vi "process.vi"() -> ()   [LabVIEW 2019]
uses:
  drivers/evcxxx.lvlib
panel:
  out "Device":T1={"Name"="---", "Type"=enum."Standard", "Class"=0, "FW-Rev"=0.0, "HV max"=0.0, "Emis max"=0.0}
  out "Data Cluster #1":T2 {"Flux" format="%^#_6e"; "Fil" format="%.2f"; "Emis" format="%.1f"; "HV" format="%#.0f"}
  out "Data Cluster #2":T3 {"Aux" format="%.2f"; "Sample" format="%^#_6e"}
  out "Data Cluster #3":T4 {"Fil max" format="%.2f"; "Emis max" format="%.1f"}
  out "Data Cluster #4":T5={"TMR Start"="00:00:00", "TMR/CLK"="00:00:00", "Dep Start"=0.0, "Dep/Exp"=0.0} {"Dep/Exp" format="%^#_6e"; "Dep Start" format="%^#_6e"}
  out "Data Cluster #5":T6 {"Fil nom" format="%.2f"; "Emis nom" format="%.1f"}
  out "Data Cluster #6":cluster{"AU-SP":dbl, "FL-SP":dbl} {"FL-SP" format="%^#_6e"; "AU-SP" format="%.2f"}
  out "Data Cluster #7":T7
  out "Status":T8
  out "Shutter":T9
  in  "OK":bool
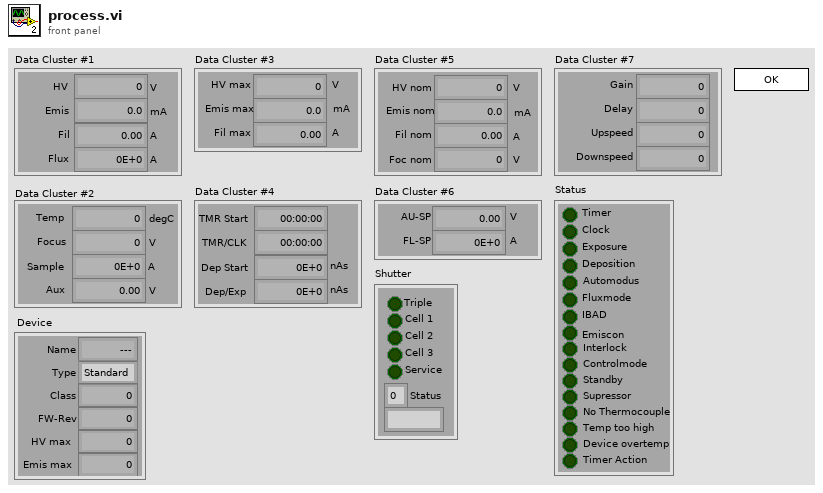
[diagram p1: front panel]
types:
  T1 = cluster{"Name":string, "Type":enum16{"Standard", "IBAD", "Supr"}, "Class":u16, "FW-Rev":dbl, "HV max":dbl, "Emis max":dbl}
  T2 = cluster{"HV":dbl, "Emis":dbl, "Fil":dbl, "Flux":dbl}
  T3 = cluster{"Temp":dbl, "Focus":dbl, "Sample":dbl, "Aux":dbl}
  T4 = cluster{"HV max":dbl, "Emis max":dbl, "Fil max":dbl}
  T5 = cluster{"TMR Start":string, "TMR/CLK":string, "Dep Start":dbl, "Dep/Exp":dbl}
  T6 = cluster{"HV nom":dbl, "Emis nom":dbl, "Fil nom":dbl, "Foc nom":dbl}
  T7 = cluster{"Gain":i32, "Delay":i32, "Upspeed":i32, "Downspeed":i32}
  T8 = cluster{"Timer":bool, "Clock":bool, "Exposure":bool, "Deposition":bool, "Automodus":bool, "Fluxmode":bool, "IBAD":bool, "Emiscon":bool, "Interlock":bool, "Controlmode":bool, "Standby":bool, "Supressor":bool, "No Thermocouple":bool, "Temp too high":bool, "Device overtemp":bool, "Timer Action":bool}
  T9 = cluster{"Triple":bool, "Cell 1":bool, "Cell 2":bool, "Cell 3":bool, "Service":bool, "iStatus":u8, "strStatus":string}
  T10 = enum32{"Invalid", "Standard", "Closed", "Hidden", "Minimized", "Maximized"}
  T11 = enum32{"invalid app kind", "Development System", "Run Time System", "Student Edition", "Embedded LabVIEW", "Evaluation", "Custom"}
  T12 = cluster{"Core":cluster{"Current VI Reference":refnum<vi>, "Close Panel on Exit?":bool}, "Your Boolean data":bool, "Your string data":string}
  T13 = cluster{"Current VI Reference":refnum<vi>, "Close Panel on Exit?":bool}
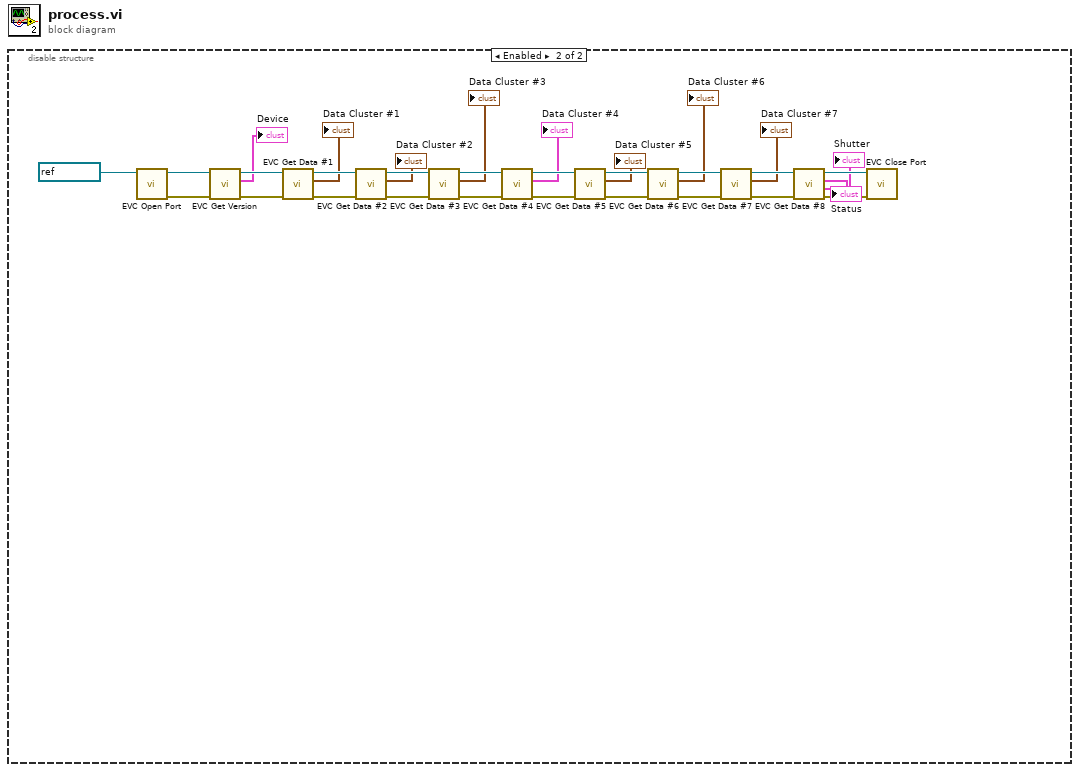
[diagram p0: block diagram]
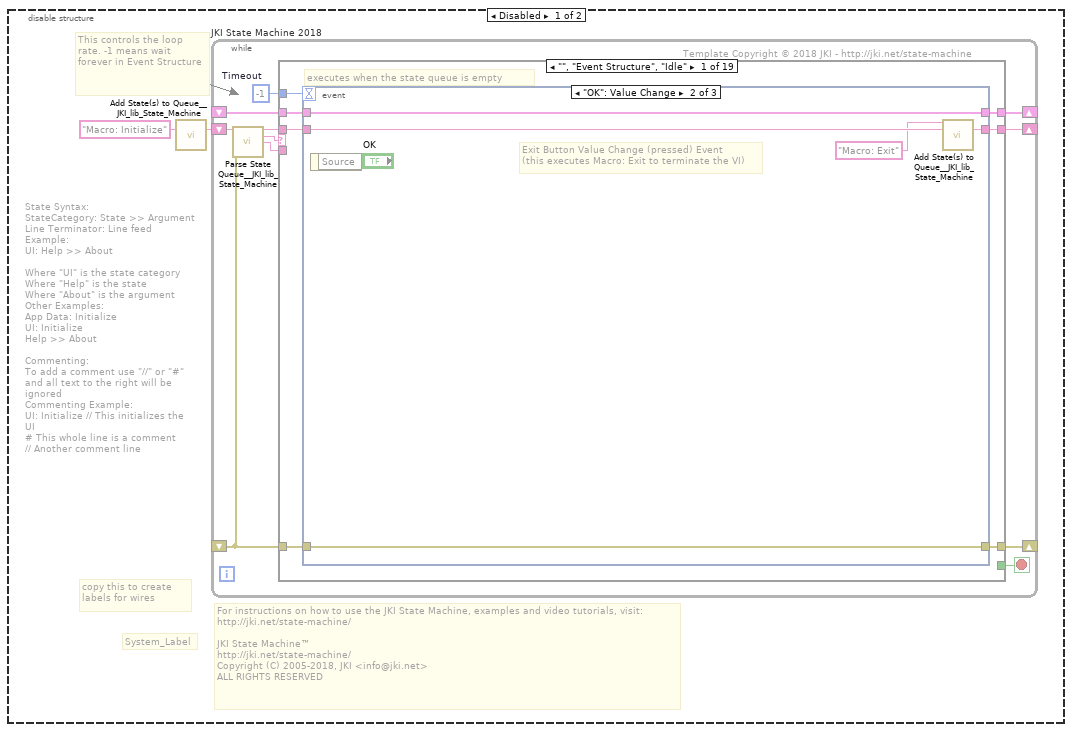
[diagram p2: hidden frame]
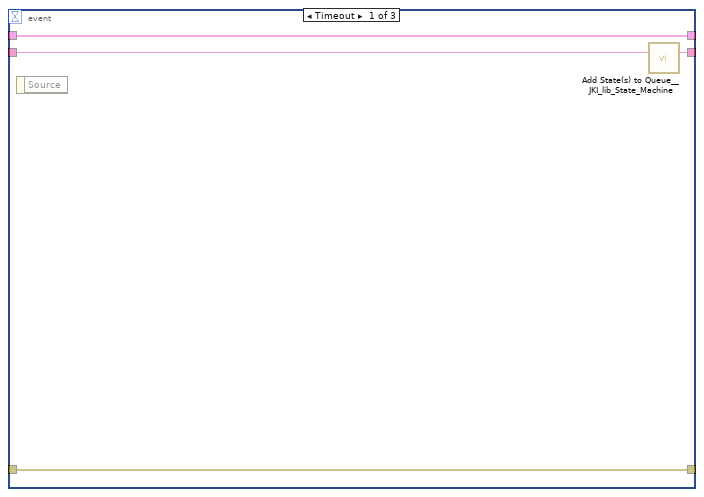
[diagram p3: hidden frame]
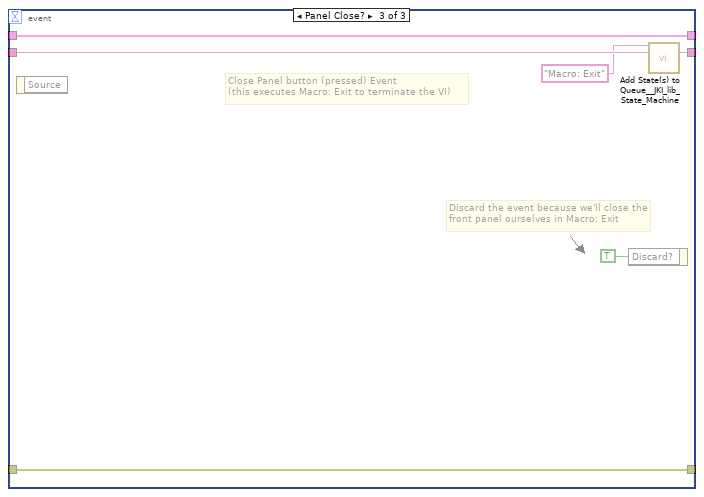
[diagram p4: hidden frame]
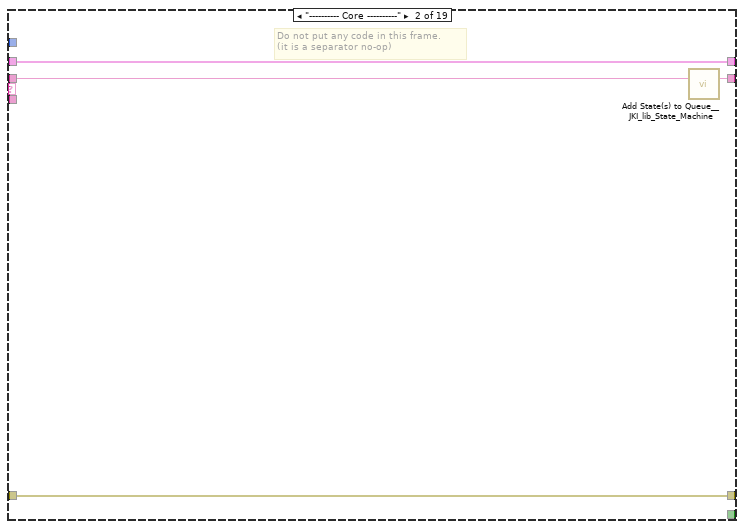
[diagram p5: hidden frame]
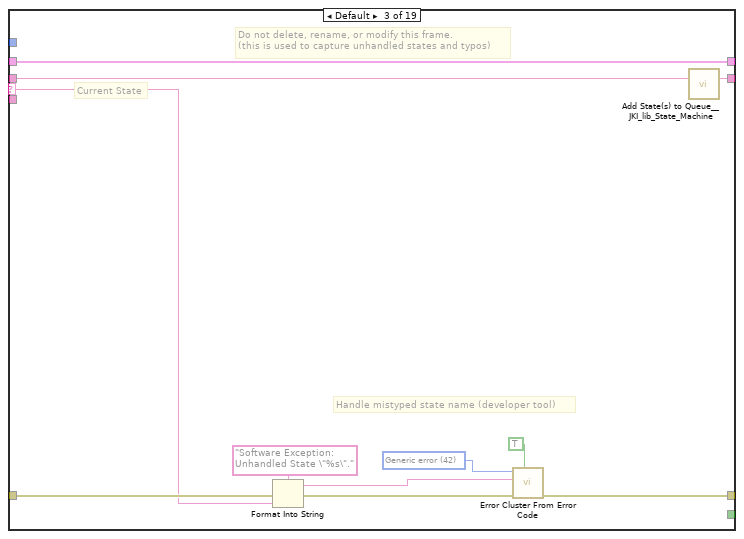
[diagram p6: hidden frame]
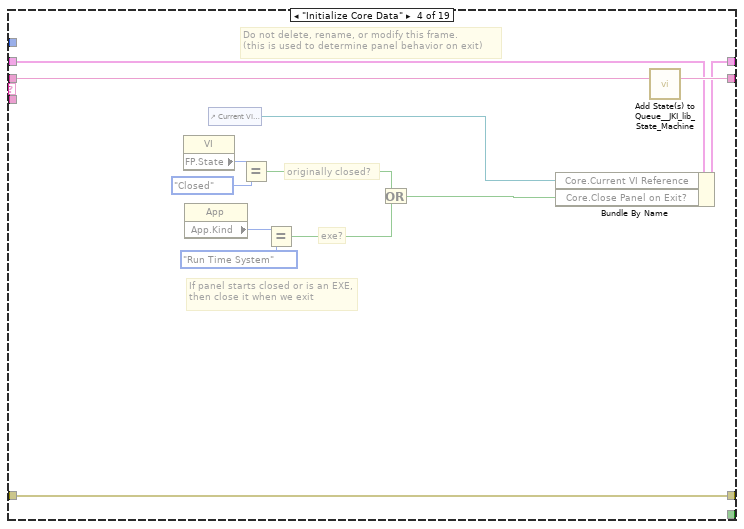
[diagram p7: hidden frame]
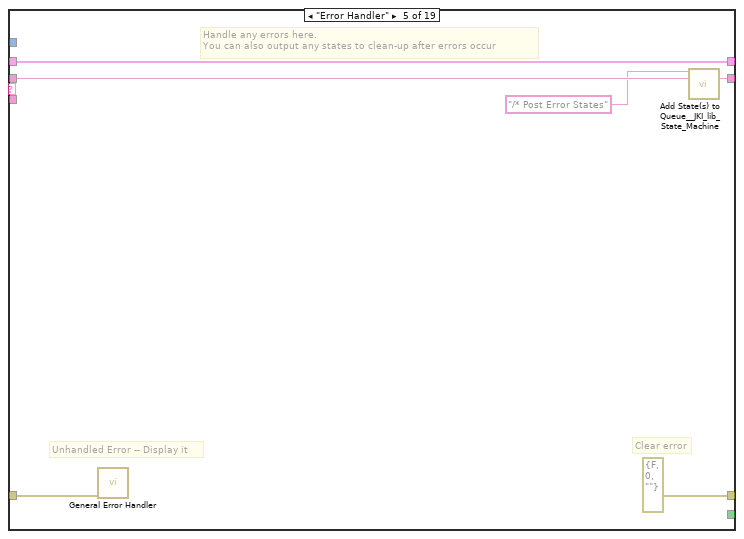
[diagram p8: hidden frame]
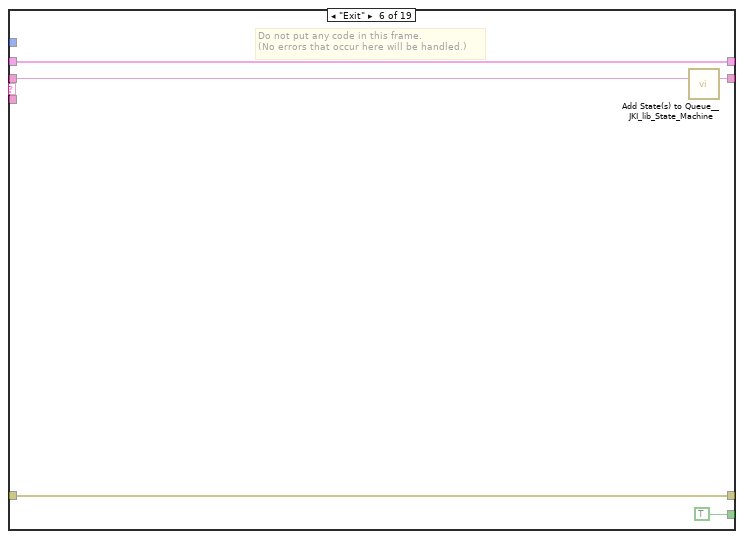
[diagram p9: hidden frame]
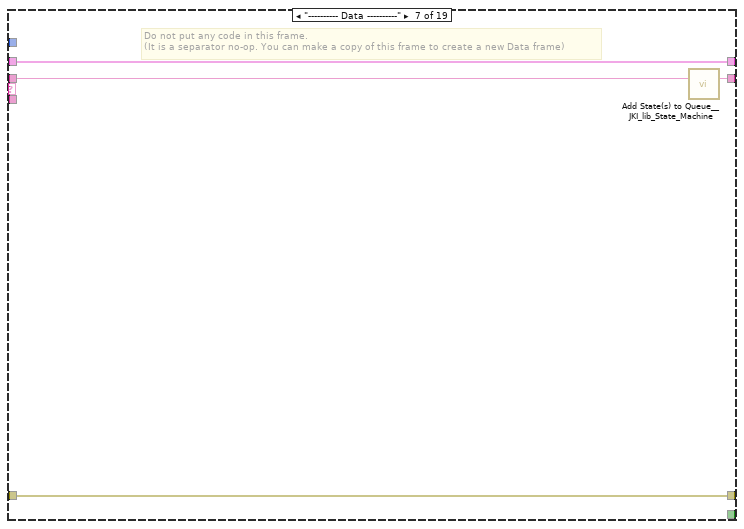
[diagram p10: hidden frame]
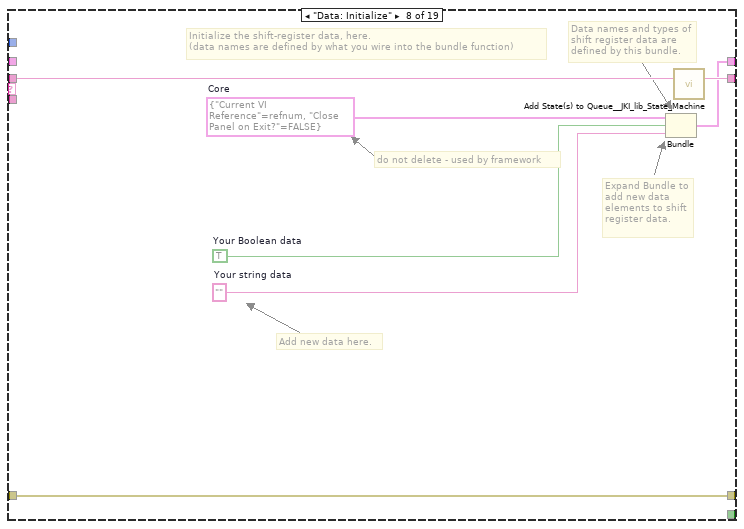
[diagram p11: hidden frame]
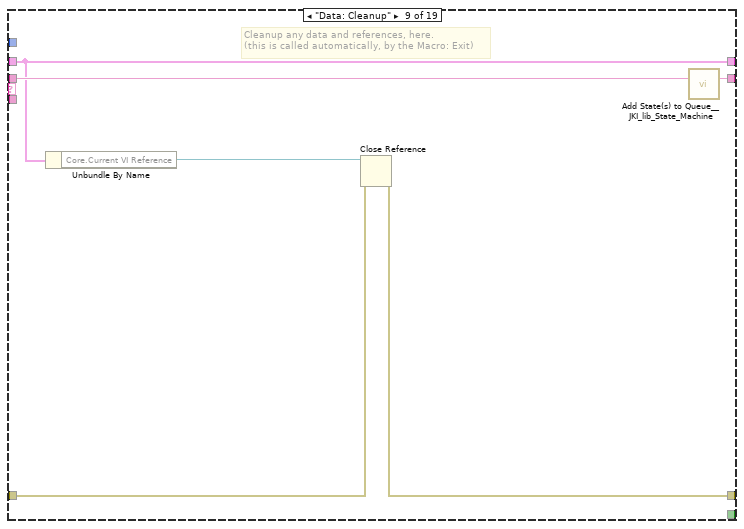
[diagram p12: hidden frame]
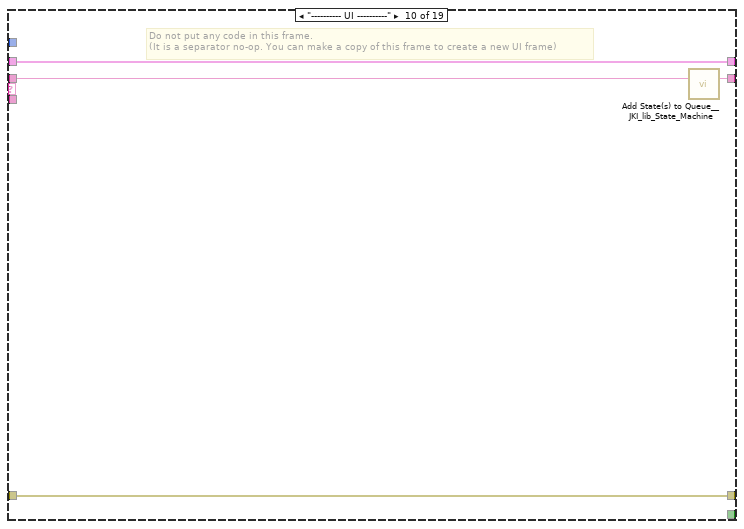
[diagram p13: hidden frame]
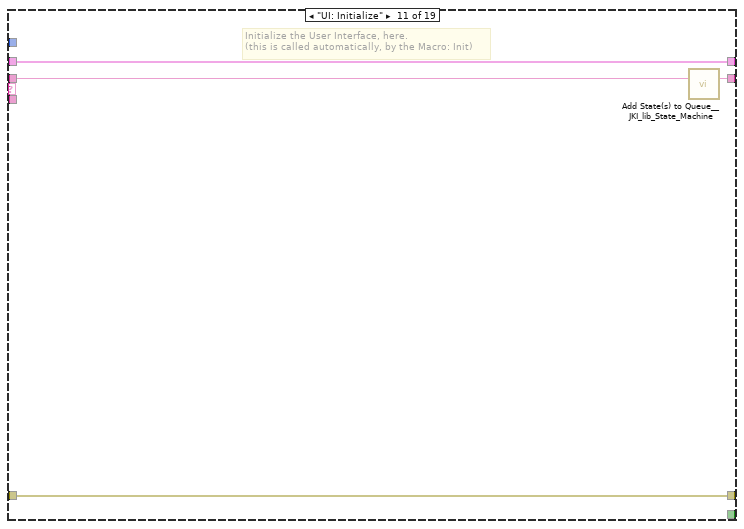
[diagram p14: hidden frame]
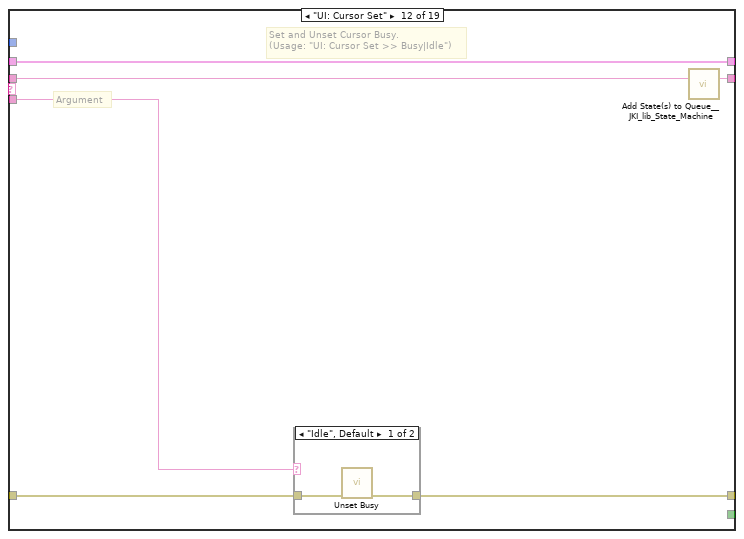
[diagram p15: hidden frame]
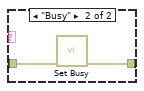
[diagram p16: hidden frame]
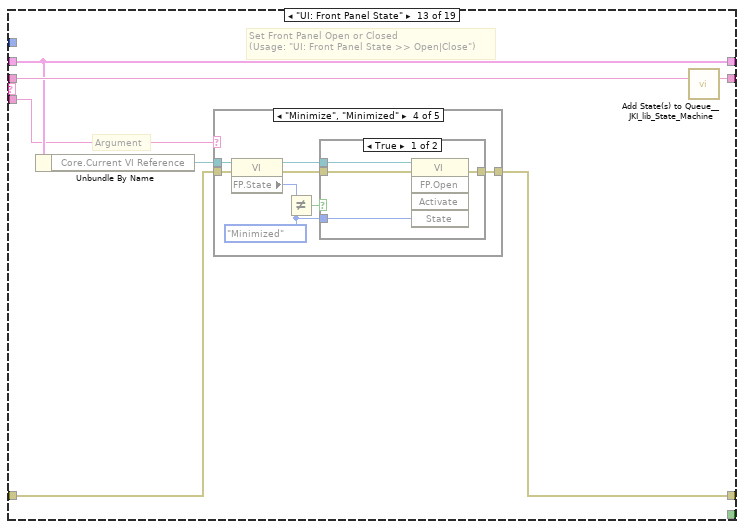
[diagram p17: hidden frame]
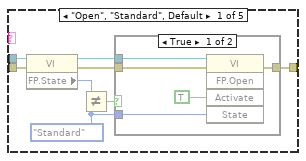
[diagram p18: hidden frame]
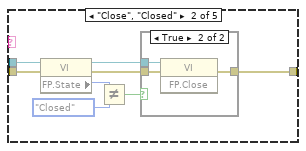
[diagram p20: hidden frame]
diagram:
  n1 = disable-structure shown="Enabled" {
    frame Disabled {
      # "For instructions on how to use the JKI State Machine, examples and video tutorials, visit:\nhttp://jki.net/state-machine/\n\nJKI State Machine™\nhttp://jki.net/state-machine/\nCopyright (C) 2005-2018, JKI <info@jki.net>\nALL RIGHTS RESERVED"
      # "State Syntax:\nStateCategory: State >> Argument\nLine Terminator: Line feed\nExample:\nUI: Help >> About\n\nWhere \"UI\" is the state category\nWhere \"Help\" is the state\nWhere \"About\" is the argument\nOther Examples:\nApp Data: Initialize\nUI: Initialize\nHelp >> About\n\nCommenting:\nTo add a comment use \"//\" or \"#\" and all text to the right will be ignored\nCommenting Example:\nUI: Initialize // This initializes the UI\n# This whole line is a comment\n// Another comment line"
      # "copy this to create labels for wires"
      # "This controls the loop rate. -1 means wait forever in Event Structure"
      # "System_Label"
      n2 = call <vilib>:"Add State(s) to Queue__JKI_lib_State_Machine.vi"("State(s) in (\"\")"="Macro: Initialize") -> ("States Out"=w2:string)  [unwired: 14 in]
      n3 = while "JKI State Machine 2018" {
        shift-right: [w6] -> _
        shift-left: _ -> [w5]
        shift-right: [w9] -> _
        shift-left: _ -> [w3]
        shift-right: [w8] -> _
        shift-left: w2 -> [w10]
        stop <- w7 stop-if-true
        w4 = -1  # Timeout
        # "Template Copyright © 2018 JKI - http://jki.net/state-machine"
        n4 = call <vilib>:"Parse State Queue__JKI_lib_State_Machine.vi"("State Queue"=w10, "Error In (no error)"=w3) -> ("Remaining States"=w12:string, "Current State"=w13:string, "Arguments"=w11:string)  [unwired: 11 in]
        n5 = case shown="\"\", \"Event Structure\", \"Idle\"" w13 {
          selector: w13 -> [_ _ w40 _ _ _ _ _ _ _ _ _ _ _ _ _ _ _ _]
          tunnel: w12 -> [w20 w39 w44 w63 w69 w74 w78 w85 w91 w95 w99 w105 w116 w185 w190 w200 w204 w208 w212]
          tunnel: w11 -> [_ _ _ _ _ _ _ _ _ _ _ w100 w110 _ _ _ _ _ _]
          tunnel: w5 -> [w18 w36 w42 w56 w66 w72 w75 _ w86 w92 w97 w103 w112 w182 w187 w197 w201 w205 w209]
          tunnel: [w17 w37 w46 w60 errorcluster {"status"=FALSE, "code"=0, "source"=""} ("error out") w71 w76 w82 w87 w93 w96 w101 w113 w183 w188 w198 w202 w206 w210] -> w9
          tunnel: w3 -> [w16 w37 w45 w60 w65 w71 w76 w82 w88 w93 w96 w102 w114 w183 w188 w198 w202 w206 w210]
          tunnel: [w19 w38 w43 w62 w68 w73 w77 w84 w90 w94 w98 w104 w115 w184 w189 w199 w203 w207 w211] -> w8
          tunnel: [_ _ _ _ _ TRUE _ _ _ _ _ _ _ _ _ _ _ _ _] -> w7
          tunnel: [w15 w36 w42 w61 w66 w72 w75 w83 w86 w92 w97 w103 w112 w182 w187 w197 w201 w205 w209] -> w6
          tunnel: w4 -> [w14 _ _ _ _ _ _ _ _ _ _ _ _ _ _ _ _ _ _]
          frame "", "Event Structure", "Idle" {
            # "executes when the state queue is empty"
            n6 = event shown="[1] \"OK\": Value Change" {
              selector: _ -> [_ _ _]
              dyn-events: _ -> [_ _ _]
              timeout: w14 -> [_ _ _]
              tunnel: w20 -> [w24 w29 w35]
              tunnel: [w23 w28 w34] -> w19
              tunnel: w18 -> [w21 w26 w32]
              tunnel: [w22 w27 w33] -> w17
              tunnel: w16 -> [w22 w27 w33]
              tunnel: [w21 w26 w32] -> w15
              event Timeout {
                n7 = event-data() -> ()  [unwired: 1 in, 1 out]
                n8 = call <vilib>:"Add State(s) to Queue__JKI_lib_State_Machine.vi"("State(s) in (\"\")"=w24) -> ("States Out"=w23:string)  [unwired: 14 in]
              }
              event "OK": Value Change {
                # "Exit Button Value Change (pressed) Event\n(this executes Macro: Exit to terminate the VI)"
                n9 = event-data() -> ()  [unwired: 1 in, 1 out]
                n10 = call <vilib>:"Add State(s) to Queue__JKI_lib_State_Machine.vi"("State(s) in Front (\"\")"="Macro: Exit", "State(s) in (\"\")"=w29) -> ("States Out"=w28:string)  [unwired: 13 in]
              }
              event Panel Close? {
                # "Discard the event because we'll close the front panel ourselves in Macro: Exit"
                # "Close Panel button (pressed) Event\n(this executes Macro: Exit to terminate the VI)"
                n11 = event-data() -> ()  [unwired: 1 in, 1 out]
                n12 = event-data("Discard?"=TRUE) -> ()  [unwired: 1 in, 1 out]
                n13 = call <vilib>:"Add State(s) to Queue__JKI_lib_State_Machine.vi"("State(s) in Front (\"\")"="Macro: Exit", "State(s) in (\"\")"=w35) -> ("States Out"=w34:string)  [unwired: 13 in]
              }
            }
          }
          frame "---------- Core ----------" {
            # "Do not put any code in this frame.\n(it is a separator no-op)"
            n14 = call <vilib>:"Add State(s) to Queue__JKI_lib_State_Machine.vi"("State(s) in (\"\")"=w39) -> ("States Out"=w38:string)  [unwired: 14 in]
          }
          frame Default {
            w49 = 42 items=["No error", "Argument error", "Memory is full", "Out of zone", "End of file", "File already open", "Generic file I/O error", "File not found", "File permission error", "Disk is full", "Duplicate path", "Too many files open", "System feature not enabled", "Resource file not found", "Cannot add resource", "Resource not found", "Image not found", "Image memory error", "Pen does not exist", "Config type invalid", "Config token not found", "Config parse error", "Config memory error", "Bad external code format", "Bad external code offset", "External code not present", "Null window", "Destroy window error", "Null menu", "Print aborted", "Bad print record", "Print driver error", "Windows error during printing", "Memory error during printing", "Print dialog error", "Generic print error", "Invalid device refnum", "Device not found", "Device parameter error", "Device unit error", "Cannot open device", "Device call aborted", "Generic error", "Cancelled by user", "Object ID too low", "Object ID too high", "Object not in heap", "Unknown heap", "Unknown object (invalid DefProc)", "Unknown object (DefProc not in table)", "Message out of range", "Invalid (null) method", "Unknown message", "Manager call not supported", "Bad address", "Network operation in progress", "Network operation timed out", "Connection is busy", "Network attribute not supported", "Network error", "Address in use", "System out of memory", "Connection aborted", "Connection refused", "Not connected", "Already connected", "Connection closed", "Initialization error (interapplication manager)", "Bad occurrence", "Wait on unbound occurrence handler", "Occurrence queue overflow", "Datalog type conflict", "Unused", "Unrecognized type (interapplication manager)", "Memory corrupt", "Failed to make temporary DLL", "Old CIN version", "Drag socket not found", "Failed to load drop-object", "Failed to register OLE object", "Failed to release OLE object", "Format specifier type mismatch", "Unknown format specifier", "Too few format specifiers", "Too many format specifiers", "Scan failed", "Newer CIN version", "Error converting to variant", "Runtime menu error", "Password tampered", "Variant attribute not found", "Incompatible variant data type", "Event data is not available", "Event Store is not present", "Occurrence is not found", "Event Queue is not created", "Event info is not available", "Refnum passed is NULL", "Error retrieving Class GUID", "Error retrieving CoClass GUID", "Error retrieving TypeLib GUID.", "Bad built application magic bytes.", "Specific driver is different from the specific driver associated with the Logical Name.", "There is no session opened to the class driver.", "Max Error", "MAX - Error with config objects", "MAX - Error loading configuration", "MAX - Group not supported"]
            # "Current State"
            # "Do not delete, rename, or modify this frame.\n(this is used to capture unhandled states and typos)"
            # "Handle mistyped state name (developer tool)"
            n15 = Format Into String(format string="Software Exception: Unhandled State \"%s\"." ("message"), error in=w45, w40) -> (resulting string=w48:string, error out=w47:errorcluster)  [unwired: 1 in]
            n16 = call <vilib>:"Error Cluster From Error Code.vi"("show call chain? (False)"=TRUE, "error in (no error)"=w47, "error message (\"\")"=w48, "error code (0)"=w49) -> ("error out"=w46:errorcluster)  [unwired: 5 in]
            n17 = call <vilib>:"Add State(s) to Queue__JKI_lib_State_Machine.vi"("State(s) in (\"\")"=w44) -> ("States Out"=w43:string)  [unwired: 14 in]
          }
          frame "Initialize Core Data" {
            # "Do not delete, rename, or modify this frame.\n(this is used to determine panel behavior on exit)"
            # "originally closed?"
            # "exe?"
            # "If panel starts closed or is an EXE, then close it when we exit"
            n18 = property class="VI"() -> ("FP.State"=w53:T10)  [unwired: 2 in, 2 out]
            n19 = property class="App"() -> ("App.Kind"=w59:T11)  [unwired: 2 in, 2 out]
            n20 = control-ref of="Current VI Reference"() -> (w54:refnum<vi>)
            n21 = Equal?(x=w53, y=T10."Closed" ("Front Panel Window:State")) -> (x = y?=w51:bool)
            n22 = Equal?(x=w59, y=T11."Run Time System" ("Application:Kind")) -> (x = y?=w57:bool)
            n23 = Or(x=w51, y=w57) -> (x .or. y?=w55:bool)
            n24 = Bundle By Name(cluster=w56, "Core.Current VI Reference"=w54, "Core.Close Panel on Exit?"=w55) -> (w61:T12)
            n25 = call <vilib>:"Add State(s) to Queue__JKI_lib_State_Machine.vi"("State(s) in (\"\")"=w63) -> ("States Out"=w62:string)  [unwired: 14 in]
          }
          frame "Error Handler" {
            # "Unhandled Error -- Display it"
            # "Handle any errors here.\nYou can also output any states to clean-up after errors occur"
            # "Clear error"
            n26 = call <vilib>:"General Error Handler.vi"("error in (no error)"=w65) -> ()  [unwired: 10 in, 5 out]
            n27 = call <vilib>:"Add State(s) to Queue__JKI_lib_State_Machine.vi"("State(s) in Front (\"\")"="/* Post Error States", "State(s) in (\"\")"=w69) -> ("States Out"=w68:string)  [unwired: 13 in]
          }
          frame "Exit" {
            # "Do not put any code in this frame.\n(No errors that occur here will be handled.)"
            n28 = call <vilib>:"Add State(s) to Queue__JKI_lib_State_Machine.vi"("State(s) in (\"\")"=w74) -> ("States Out"=w73:string)  [unwired: 14 in]
          }
          frame "---------- Data ----------" {
            # "Do not put any code in this frame.\n(It is a separator no-op. You can make a copy of this frame to create a new Data frame)"
            n29 = call <vilib>:"Add State(s) to Queue__JKI_lib_State_Machine.vi"("State(s) in (\"\")"=w78) -> ("States Out"=w77:string)  [unwired: 14 in]
          }
          frame "Data: Initialize" {
            w79 = T13 {"Current VI Reference"=refnum, "Close Panel on Exit?"=FALSE}  # Core
            w81 = TRUE  # Your Boolean data
            w80 = ""  # Your string data
            # "do not delete - used by framework"
            # "Expand Bundle to add new data elements to shift register data."
            # "Add new data here."
            # "Data names and types of shift register data are defined by this bundle."
            # "Initialize the shift-register data, here.\n(data names are defined by what you wire into the bundle function)"
            n30 = Bundle("Core"=w79, "Your Boolean data"=w81, "Your string data"=w80) -> (w83:T12)  [unwired: 1 in]
            n31 = call <vilib>:"Add State(s) to Queue__JKI_lib_State_Machine.vi"("State(s) in (\"\")"=w85) -> ("States Out"=w84:string)  [unwired: 14 in]
          }
          frame "Data: Cleanup" {
            # "Cleanup any data and references, here.\n(this is called automatically, by the Macro: Exit)"
            n32 = Unbundle By Name(w86) -> ("Core.Current VI Reference"=w89:refnum<vi>)
            n33 = Close Reference(reference=w89, error in (no error)=w88) -> (error out=w87:errorcluster)
            n34 = call <vilib>:"Add State(s) to Queue__JKI_lib_State_Machine.vi"("State(s) in (\"\")"=w91) -> ("States Out"=w90:string)  [unwired: 14 in]
          }
          frame "---------- UI ----------" {
            # "Do not put any code in this frame.\n(It is a separator no-op. You can make a copy of this frame to create a new UI frame)"
            n35 = call <vilib>:"Add State(s) to Queue__JKI_lib_State_Machine.vi"("State(s) in (\"\")"=w95) -> ("States Out"=w94:string)  [unwired: 14 in]
          }
          frame "UI: Initialize" {
            # "Initialize the User Interface, here.\n(this is called automatically, by the Macro: Init)"
            n36 = call <vilib>:"Add State(s) to Queue__JKI_lib_State_Machine.vi"("State(s) in (\"\")"=w99) -> ("States Out"=w98:string)  [unwired: 14 in]
          }
          frame "UI: Cursor Set" {
            # "Argument"
            # "Set and Unset Cursor Busy.\n(Usage: \"UI: Cursor Set >> Busy|Idle\")"
            n37 = case shown="\"Idle\", Default" w100 {
              tunnel: w102 -> [w107 w109]
              tunnel: [w106 w108] -> w101
              frame "Idle", Default {
                n38 = call <vilib>:"Unset Busy.vi"("error in (no error)"=w107) -> ("error out"=w106:errorcluster)  [unwired: 10 in]
              }
              frame "Busy" {
                n39 = call <vilib>:"Set Busy.vi"("error in (no error)"=w109) -> ("error out"=w108:errorcluster)  [unwired: 9 in, 1 out]
              }
            }
            n40 = call <vilib>:"Add State(s) to Queue__JKI_lib_State_Machine.vi"("State(s) in (\"\")"=w105) -> ("States Out"=w104:string)  [unwired: 14 in]
          }
          frame "UI: Front Panel State" {
            # "Argument"
            # "Set Front Panel Open or Closed\n(Usage: \"UI: Front Panel State >> Open|Close\")"
            n41 = Unbundle By Name(w112) -> ("Core.Current VI Reference"=w111:refnum<vi>)
            n42 = case shown="\"Minimize\", \"Minimized\"" w110 {
              tunnel: w114 -> [w122 w137 w148 w161 w174]
              tunnel: [w124 w138 w150 w163 w176] -> w113
              tunnel: w111 -> [w123 w135 w149 w162 w175]
              frame "Open", "Standard", Default {
                w117 = T10."Standard" ("State")
                n43 = property class="VI"(reference=w123, error in=w122) -> (reference out=w120:refnum<vi>, error out=w121:errorcluster, "FP.State"=w119:T10)
                n44 = Not Equal?(x=w119, y=w117) -> (x != y?=w118:bool)
                n45 = case shown="True" w118 {
                  tunnel: [w128 w130] -> w124
                  tunnel: w121 -> [w127 w130]
                  tunnel: w120 -> [w126 _]
                  tunnel: w117 -> [w125 _]
                  frame True {
                    n46 = invoke class="VI" method="FP.Open"(reference=w126, error in=w127, "Activate"=TRUE, "State"=w125) -> (error out=w128:errorcluster)  [unwired: 1 in, 4 out]
                  }
                  frame False {
                  }
                }
              }
              frame "Close", "Closed" {
                n47 = property class="VI"(reference=w135, error in=w137) -> (reference out=w134:refnum<vi>, error out=w136:errorcluster, "FP.State"=w132:T10)
                n48 = Not Equal?(x=w132, y=T10."Closed" ("Front Panel Window:State")) -> (x != y?=w131:bool)
                n49 = case shown="True" w131 {
                  tunnel: [w139 w142] -> w138
                  tunnel: w136 -> [w139 w141]
                  tunnel: w134 -> [_ w140]
                  frame False {
                  }
                  frame True {
                    n50 = invoke class="VI" method="FP.Close"(reference=w140, error in=w141) -> (error out=w142:errorcluster)  [unwired: 1 in, 2 out]
                  }
                }
              }
              frame "Hidden", "Hide" {
                w143 = T10."Hidden" ("State")
                n51 = property class="VI"(reference=w149, error in=w148) -> (reference out=w146:refnum<vi>, error out=w147:errorcluster, "FP.State"=w145:T10)
                n52 = Not Equal?(x=w145, y=w143) -> (x != y?=w144:bool)
                n53 = case shown="True" w144 {
                  tunnel: [w154 w155] -> w150
                  tunnel: w147 -> [w153 w155]
                  tunnel: w146 -> [w152 _]
                  tunnel: w143 -> [w151 _]
                  frame True {
                    n54 = invoke class="VI" method="FP.Open"(reference=w152, error in=w153, "State"=w151) -> (error out=w154:errorcluster)  [unwired: 2 in, 4 out]
                  }
                  frame False {
                  }
                }
              }
              frame "Minimize", "Minimized" {
                w156 = T10."Minimized" ("State")
                n55 = property class="VI"(reference=w162, error in=w161) -> (reference out=w159:refnum<vi>, error out=w160:errorcluster, "FP.State"=w158:T10)
                n56 = Not Equal?(x=w158, y=w156) -> (x != y?=w157:bool)
                n57 = case shown="True" w157 {
                  tunnel: [w167 w168] -> w163
                  tunnel: w160 -> [w166 w168]
                  tunnel: w159 -> [w165 _]
                  tunnel: w156 -> [w164 _]
                  frame True {
                    n58 = invoke class="VI" method="FP.Open"(reference=w165, error in=w166, "State"=w164) -> (error out=w167:errorcluster)  [unwired: 2 in, 4 out]
                  }
                  frame False {
                  }
                }
              }
              frame "Maximize", "Maximized" {
                w169 = T10."Maximized" ("State")
                n59 = property class="VI"(reference=w175, error in=w174) -> (reference out=w172:refnum<vi>, error out=w173:errorcluster, "FP.State"=w171:T10)
                n60 = Not Equal?(x=w171, y=w169) -> (x != y?=w170:bool)
                n61 = case shown="True" w170 {
                  tunnel: [w180 w181] -> w176
                  tunnel: w173 -> [w179 w181]
                  tunnel: w172 -> [w178 _]
                  tunnel: w169 -> [w177 _]
                  frame True {
                    n62 = invoke class="VI" method="FP.Open"(reference=w178, error in=w179, "State"=w177) -> (error out=w180:errorcluster)  [unwired: 2 in, 4 out]
                  }
                  frame False {
                  }
                }
              }
            }
            n63 = call <vilib>:"Add State(s) to Queue__JKI_lib_State_Machine.vi"("State(s) in (\"\")"=w116) -> ("States Out"=w115:string)  [unwired: 14 in]
          }
          frame "---------- Macro ----------" {
            # "Do not put any code in this frame.\n(It is a separator no-op. You can make a copy of this frame to create a new Macro frame)"
            n64 = call <vilib>:"Add State(s) to Queue__JKI_lib_State_Machine.vi"("State(s) in (\"\")"=w185) -> ("States Out"=w184:string)  [unwired: 14 in]
          }
          frame "Macro: Initialize" {
            w186 = "Data: Initialize\nInitialize Core Data\nUI: Initialize\nUI: Front Panel State >> Open"  # Data: Initialize Initialize Core Data UI: Initialize UI: Front Panel State >> Open
            # "Initialization Macro\n(This is called once, when the VI starts)"
            n65 = call <vilib>:"Add State(s) to Queue__JKI_lib_State_Machine.vi"("State(s) in Front (\"\")"=w186, "State(s) in (\"\")"=w190) -> ("States Out"=w189:string)  [unwired: 13 in]
          }
          frame "Macro: Exit" {
            # "Exit Macro\n(This is called once, when the VI exits)"
            n66 = Unbundle By Name(w197) -> ("Core.Close Panel on Exit?"=w196:bool)
            n67 = Select(t="UI: Front Panel State >> Close", s=w196, f="") -> (s? t:f=w193:string)
            n68 = call <vilib>:"Add State(s) to Queue__JKI_lib_State_Machine.vi"("State(s) in (\"\")"=w193, "State(s) at Back (\"\")"="Data: Cleanup\nExit") -> ("States Out"=w191:string)  [unwired: 13 in]
            n69 = call <vilib>:"Add State(s) to Queue__JKI_lib_State_Machine.vi"("State(s) in Front (\"\")"=w191, "State(s) in (\"\")"=w200) -> ("States Out"=w199:string)  [unwired: 13 in]
          }
          frame "---------- New Category ----------" {
            # "Template Separator\n(You can make a copy of, or modify, this frame)"
            n70 = call <vilib>:"Add State(s) to Queue__JKI_lib_State_Machine.vi"("State(s) in (\"\")"=w204) -> ("States Out"=w203:string)  [unwired: 14 in]
          }
          frame "New Category: 1" {
            # "Your code here.\n(You can make a copy of, or modify, this frame)"
            n71 = call <vilib>:"Add State(s) to Queue__JKI_lib_State_Machine.vi"("State(s) in (\"\")"=w208) -> ("States Out"=w207:string)  [unwired: 14 in]
          }
          frame "New Category: 2" {
            # "Your code here.\n(You can make a copy of, or modify, this frame)"
            n72 = call <vilib>:"Add State(s) to Queue__JKI_lib_State_Machine.vi"("State(s) in (\"\")"=w212) -> ("States Out"=w211:string)  [unwired: 14 in]
          }
        }
      }
    }
    frame Enabled {
      n73 = call "EVC Open Port.vi"("VISA ressourcen name"=refnum<visa-resource-name> "COM7") -> ("error out"=w241:errorcluster, "duplicate VISA resource name"=w242:refnum<visa-resource-name>)  [unwired: 4 in, 1 out]
      n74 = call "EVC Get Version.vi"("error in (no error)"=w241, "VISA session"=w242) -> ("error out"=w239:errorcluster, "Device"=→"Device":T1, "dup VISA session"=w240:refnum<visa-resource-name>)  [unwired: 3 in]
      n75 = call "EVC Get Data #1.vi"("error in (no error)"=w239, "VISA session"=w240) -> ("error out"=w237:errorcluster, "Data Cluster #1"=→"Data Cluster #1":T2, "dup VISA session"=w238:refnum<visa-resource-name>)  [unwired: 3 in]
      n76 = call "EVC Get Data #2.vi"("error in (no error)"=w237, "VISA session"=w238) -> ("error out"=w235:errorcluster, "Data Cluster #2"=→"Data Cluster #2":T3, "dup VISA session"=w236:refnum<visa-resource-name>)  [unwired: 3 in]
      n77 = call "EVC Get Data #3.vi"("error in (no error)"=w235, "VISA session"=w236) -> ("error out"=w233:errorcluster, "Data Cluster #3"=→"Data Cluster #3":T4, "dup VISA session"=w234:refnum<visa-resource-name>)  [unwired: 3 in]
      n78 = call "EVC Get Data #4.vi"("error in (no error)"=w233, "VISA session"=w234) -> ("error out"=w231:errorcluster, "Data Cluster #4"=→"Data Cluster #4":T5, "dup VISA session"=w232:refnum<visa-resource-name>)  [unwired: 3 in]
      n79 = call "EVC Get Data #5.vi"("error in (no error)"=w231, "VISA session"=w232) -> ("error out"=w229:errorcluster, "Data Cluster #5"=→"Data Cluster #5":T6, "dup VISA session"=w230:refnum<visa-resource-name>)  [unwired: 3 in]
      n80 = call "EVC Get Data #6.vi"("error in (no error)"=w229, "VISA session"=w230) -> ("error out"=w227:errorcluster, "Data Cluster #6"=→"Data Cluster #6":cluster{"AU-SP":dbl, "FL-SP":dbl}, "dup VISA session"=w228:refnum<visa-resource-name>)  [unwired: 3 in]
      n81 = call "EVC Get Data #7.vi"("error in (no error)"=w227, "VISA session"=w228) -> ("error out"=w225:errorcluster, "Data Cluster #7"=→"Data Cluster #7":T7, "dup VISA session"=w226:refnum<visa-resource-name>)  [unwired: 3 in]
      n82 = call "EVC Get Data #8.vi"("error in (no error)"=w225, "VISA session"=w226) -> ("error out"=w223:errorcluster, "Shutter"=→"Shutter":T9, "Status"=→"Status":T8, "dup VISA session"=w224:refnum<visa-resource-name>)  [unwired: 2 in]
      n83 = call "EVC Close Port.vi"("error in (no error)"=w223, "VISA session"=w224) -> ()  [unwired: 5 in, 1 out]
    }
  }
